vi "How to generate quadratic waveform.vi"() -> ()   [LabVIEW 2020]
panel:
  out "Waveform Graph":dbl[](graph)
  in  "C":dbl
  in  "B":dbl
  in  "A":dbl
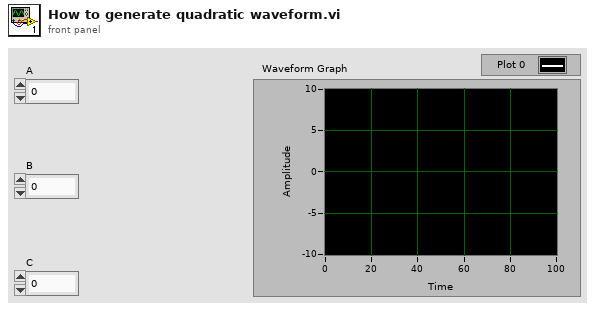
[diagram p1: front panel]
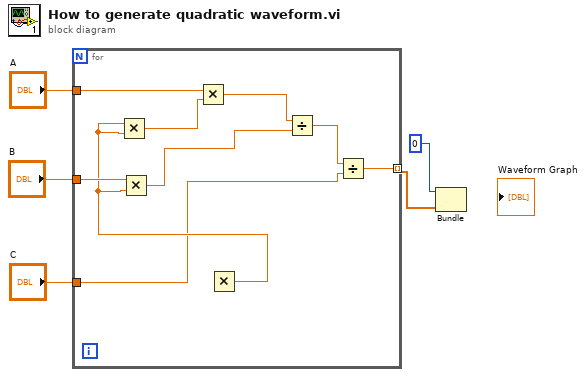
[diagram p0: block diagram]
diagram:
  n1 = for {
    tunnel: "A" -> [w14]
    tunnel: "B" -> [w9]
    tunnel: "C" -> [w7]
    tunnel: [w10] -> w1 mode=indexing
    n2 = Multiply() -> (x*y=w8:dbl)  [unwired: 2 in]
    n3 = Multiply(x=w8, y=w8) -> (x*y=w13:dbl)
    n4 = Multiply(x=w9, y=w8) -> (x*y=w6:dbl)
    n5 = Multiply(x=w14, y=w13) -> (x*y=w12:dbl)
    n6 = Divide(x=w12, y=w6) -> (x/y=w11:dbl)
    n7 = Divide(x=w11, y=w7) -> (x/y=w10:dbl)
  }
  n8 = Bundle(0, w1) -> ()  [unwired: 2 in, 1 out]
